vi "Get Pixel (Grey).vi"(4 "Error":string, 5 "Y":i32, 6 "X":i32, 7 "Image":T1={"Image ID"=0, "Channel ID"=-1}) -> (0 "Error":string, 1 "Value":u8, 3 "Image":T1={"Image ID"=0, "Channel ID"=-1})   [LabVIEW 2011, in "labvvis.lvlib"]
doc: "Retrieves the value of the pixel in Image, at the position (X, Y). This VI is applicable for both grey-scale images and single-channel images (like Red channel, Green channel and so on)."
uses:
  <userlib>/labvvis/labvvis.lvlib
  <userlib>/labvvis/VVIS Image.ctl
  labvvis.framework
panel:
  in  "Value":u8
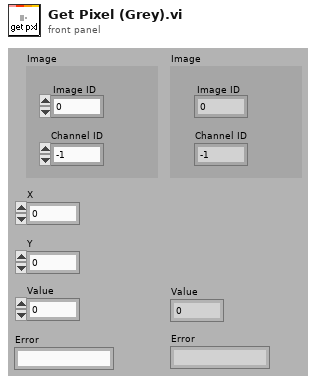
[diagram p1: front panel]
types:
  T1 = typedef "labvvis.lvlib/VVIS Image.ctl" = cluster{"Image ID":i16, "Channel ID":i16}
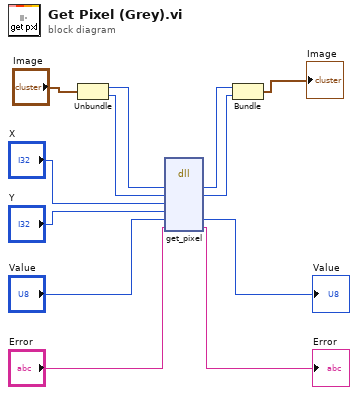
[diagram p0: block diagram]
diagram:
  n1 = Unbundle("Image") -> ("Image ID"=w11:i16, "Channel ID"=w6:i16)
  n2 = dll-call lib="labvvis.framework" fn="get_pixel"("out"=w11, "cid"=w6, "x"="X", "y"="Y", "value"="Value", "error"="Error") -> ("out"=w10:i16, "cid"=w5:i16, "value"=→"Value":u8, "error"=→"Error":string)  [unwired: 6 in, 2 out]
  n3 = Bundle("out"=w10, "cid"=w5) -> (→"Image":cluster{"out":i16, "cid":i16})  [unwired: 1 in]
